vi "putValToComplexNumByRef.vi"(8 "error in (no error)":errorcluster) -> (0 "error out":errorcluster)   [LabVIEW 2018]
doc: "Put the value into complex number by reference."
panel:
  in  "imag":dbl
  in  "real":dbl
  out "Control Value:Get 3":variant
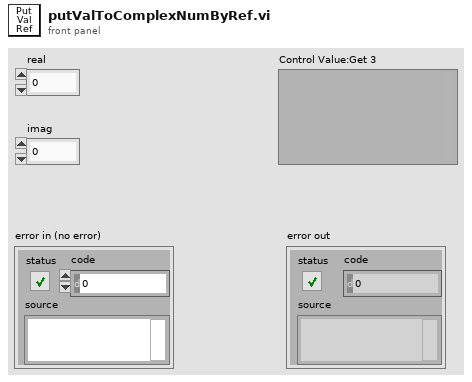
[diagram p1: front panel]
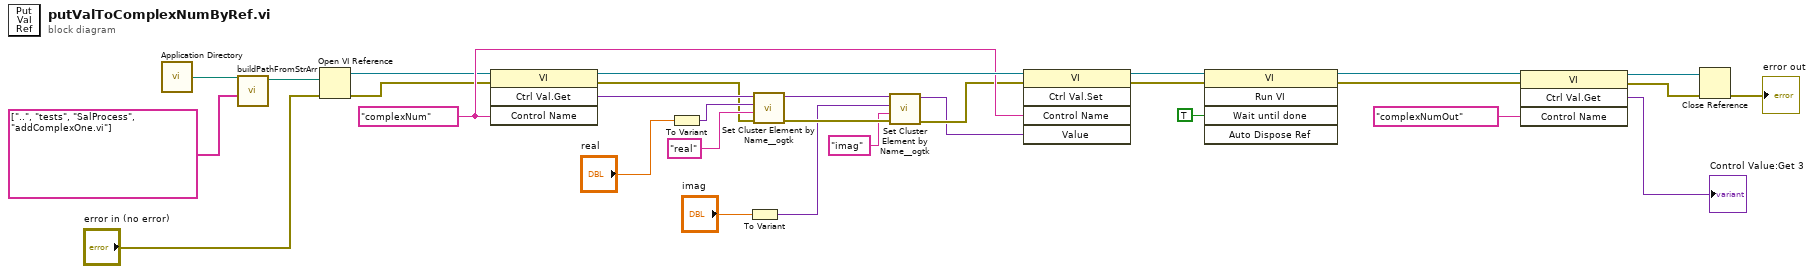
[diagram p0: block diagram]
diagram:
  w17 = "complexNum"
  n1 = call <vilib>:"Application Directory.vi"() -> ("Application Directory"=w16:path)
  n2 = call "buildPathFromStrArr.vi"("String Array"=string[] ["..", "tests", "SalProcess", "addComplexOne.vi"], "Root Path"=w16) -> ("Absolute Path"=w14:path)  [unwired: 9 in]
  n3 = Open VI Reference(vi path=w14, error in (no error)="error in (no error)") -> (vi reference=w13:refnum<vi>, error out=w12:errorcluster)  [unwired: 4 in]
  n4 = invoke class="VI" method="Ctrl Val.Get"(reference=w13, error in=w12, "Control Name"=w17) -> (reference out=w20:refnum<vi>, error out=w8:errorcluster, "Get Control Value Variant"=w10:variant)  [unwired: 1 in, 1 out]
  n5 = To Variant(anything="real") -> (Variant=w22:variant)
  n6 = To Variant(anything="imag") -> (Variant=w3:variant)
  n7 = call <userlib>:"Set Cluster Element by Name__ogtk.vi"("error in (no error)"=w8, "Element Name (\"\": New Element Data Name)"="real", "New Element Value"=w22, "Cluster"=w10) -> ("error out"=w6:errorcluster, "VCluster out"=w7:variant)  [unwired: 5 in, 1 out]
  n8 = call <userlib>:"Set Cluster Element by Name__ogtk.vi"("error in (no error)"=w6, "Element Name (\"\": New Element Data Name)"="imag", "New Element Value"=w3, "Cluster"=w7) -> ("error out"=w5:errorcluster, "VCluster out"=w1:variant)  [unwired: 5 in, 1 out]
  n9 = invoke class="VI" method="Ctrl Val.Set"(reference=w20, error in=w5, "Control Name"=w17, "Value"=w1) -> (reference out=w19:refnum<vi>, error out=w18:errorcluster)  [unwired: 1 in, 3 out]
  n10 = invoke class="VI" method="Run VI"(reference=w19, error in=w18, "Wait until done"=TRUE ("Wait Until Done")) -> (reference out=w29:refnum<vi>, error out=w28:errorcluster)  [unwired: 2 in, 3 out]
  n11 = invoke class="VI" method="Ctrl Val.Get"(reference=w29, error in=w28, "Control Name"="complexNumOut") -> (reference out=w25:refnum<vi>, error out=w24:errorcluster, "Get Control Value Variant"=→"Control Value:Get 3":variant)  [unwired: 1 in, 1 out]
  n12 = Close Reference(reference=w25, error in (no error)=w24) -> (error out=→"error out":errorcluster)
